vi "Actor Core.vi"(8 "error in":errorcluster, 11 "Main Display in":refnum<class "Main Display.lvclass">) -> (0 "error out":errorcluster, 3 "Actor out":refnum<class "Actor.lvclass">)   [LabVIEW 2016, in "Assert API Components.lvlib" / "Assert Display.lvlib" / "Main Display.lvlib" / "Main Display.lvclass"]
doc: "(<B>Filename</B>: Actor Framework.lvlib:Actor.lvclass:Actor Core.vi)\n\nReceives messages to the actor, reacts to them, and initiates any error handling that may shut the actor down.\n\nDescendant classes may override this VI to append parallel tasks for the actor to complete while it handles messages. Overrides use the Call Parent Method node."
uses:
  Main Display.lvclass
  C:/Program Files (x86)/National Instruments/LabVIEW 2016/vi.lib/ActorFramework/Actor/Actor.lvclass
  D:/Work/Projects/actor_assert_api/Base UI Component/Base UI Component/Base UI Component.lvclass
  D:/Work/Projects/actor_assert_api/Base UI Actor/Base UI Actor/Base UI Actor.lvclass
  <vilib>/ActorFramework/Actor/Actor.lvclass
  Timing Engine/Timing Engine/Timing Engine.lvclass
  Main Display.lvclass/Main Display.ctl
  Base UI Actor/Base UI Actor/Base UI Actor.lvclass/Base UI Actor.ctl
  Base UI Component/Base UI Component/Base UI Component.lvclass/Base UI Component.ctl
  <vilib>/ActorFramework/Actor/Actor.lvclass/Actor.ctl
  <vilib>/ActorFramework/Message Enqueuer/Message Enqueuer.lvclass/Message Enqueuer.ctl
  Action Configuration.ctl
  Actions.ctl
  Main Display Messages/Do Action Msg/Do Action Msg.lvclass/Do Action Msg.ctl
  <vilib>/ActorFramework/Message Enqueuer/Init from Existing Queue.vi
  <vilib>/ActorFramework/Message Enqueuer/Enqueue.vi
  Main Display Messages/Do Action Msg/Do Action Msg.lvclass
  C:/Program Files (x86)/National Instruments/LabVIEW 2016/vi.lib/ActorFramework/Message/Message.lvclass
  <vilib>/Utility/LVClass/Get LV Class Name.vi
  <resource>/AFDebug/Generate Trace for Message.vi
  <vilib>/ActorFramework/Message Priority Queue/Priority Enqueue.vi
  <vilib>/ActorFramework/Message Enqueuer/Message Enqueuer.lvclass
  Base UI Component/Base UI Component/Base UI Component.lvclass
  Right Click Menu Actions/RCM_Actions.lvclass
  Base UI Actor/Base UI Actor/Base UI Actor.lvclass
panel:
  in  "Settings":bool
  in  "Main":bool
  out "Tab Control":enum32{"Display", "Settings"}(tab)
  in  "Assert Display Data":i32(listbox)
  in  "Display Update Period":i32(slide)=1000 min=10 max=10000 scale=10.0..10000.0
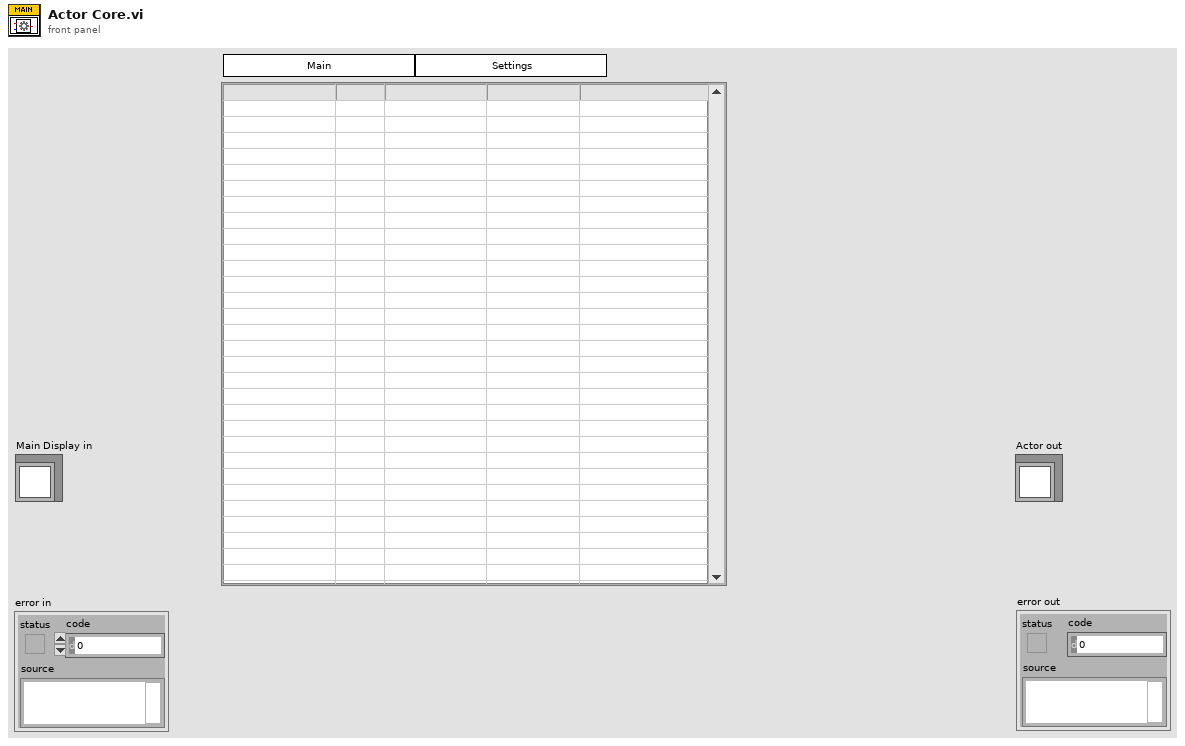
[diagram p1: front panel]
types:
  T1 = typedef "Assert API Components.lvlib/Assert Display.lvlib/Main Display.lvlib/Main Display.lvclass/Actions.ctl" = enum16{"Update Column Headers", "Update Timeout"}
  T2 = typedef "Assert API Components.lvlib/Assert Display.lvlib/Main Display.lvlib/Main Display.lvclass/Action Configuration.ctl" = cluster{"Action":T1, "Configuration":variant}
  T3 = typedef "LVPoint32TypeDef.ctl" = cluster{"Horizontal":i32, "Vertical":i32}
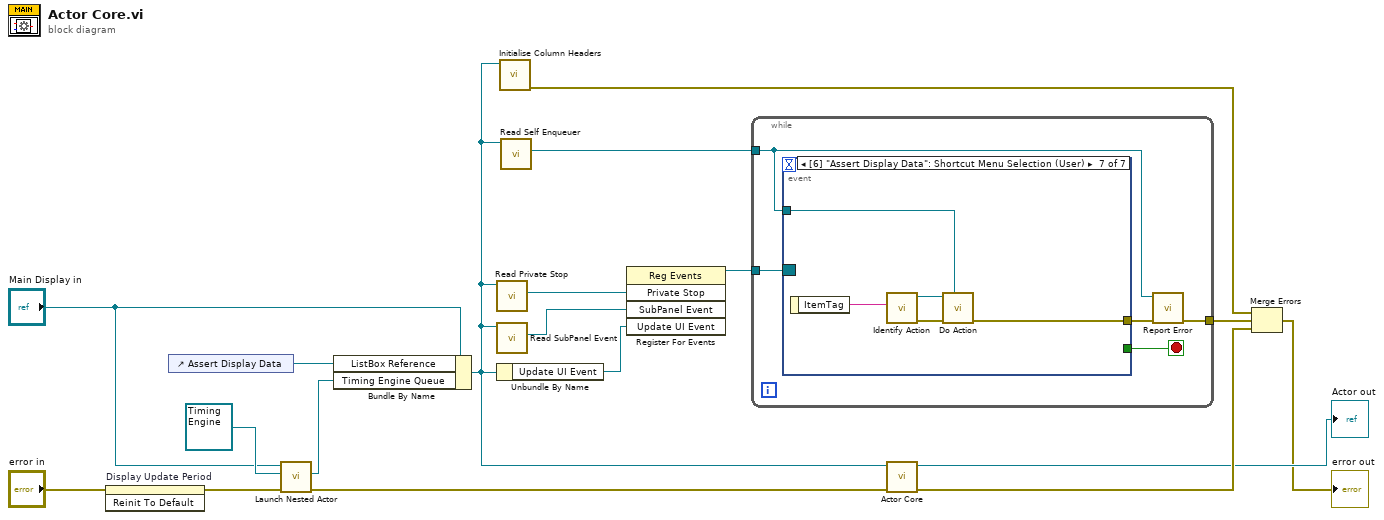
[diagram p0: block diagram]
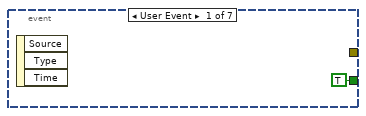
[diagram p2: hidden frame]
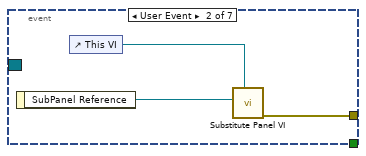
[diagram p3: hidden frame]
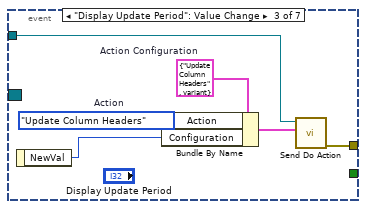
[diagram p4: hidden frame]
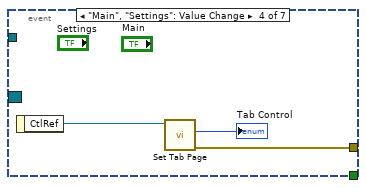
[diagram p5: hidden frame]
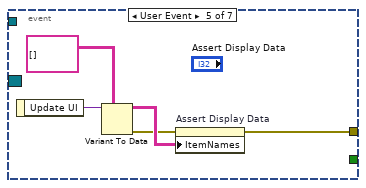
[diagram p6: hidden frame]
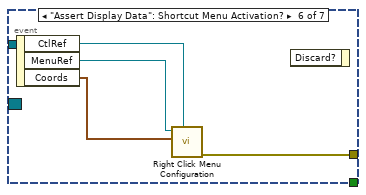
[diagram p7: hidden frame]
diagram:
  n1 = invoke on="Display Update Period" class="Slide (strict)" method="Reinit To Default"(error in="error in") -> (error out=w5:errorcluster)  [unwired: 2 in, 2 out]
  n2 = control-ref of="Assert Display Data"() -> (w1:refnum<vi>)
  n3 = call <vilib>:"Launch Nested Actor.vi"("error in (no error)"=w5, "Nested Actor"=refnum<class "Timing Engine.lvclass"> refnum ("Assert Display.lvlib:Timing Engine.lvlib:Timing Engine.lvclass"), "Caller Actor in"="Main Display in") -> ("error out"=w9:errorcluster, "Nested Actor's Enqueuer"=w10:refnum<class "Message Enqueuer.lvclass">)  [unwired: 6 in, 1 out]
  n4 = Bundle By Name(cluster="Main Display in", "ListBox Reference"=w1, "Timing Engine Queue"=w10) -> (w3:refnum<class "Main Display.lvclass">)
  n5 = call "Read Private Stop.vi"("Base UI Actor in"=w3) -> ("Private Stop"=w16:refnum<user-event>)  [unwired: 10 in]
  n6 = call "Read SubPanel Event.vi"("Base UI Component in"=w3) -> ("SubPanel Event"=w15:refnum<user-event>)  [unwired: 10 in]
  n7 = Unbundle By Name(w3) -> ("Update UI Event"=w6:refnum<user-event>)
  n8 = call "Initialise Column Headers.vi"("Main Display in"=w3) -> ("error out"=w2:errorcluster)  [unwired: 10 in]
  n9 = call <vilib>:"Read Self Enqueuer.vi"("Actor"=w3) -> ("Self Enqueuer"=w4:refnum<class "Message Enqueuer.lvclass">)  [unwired: 10 in]
  n10 = register-events(w16, w15, w6) -> (reference out=w14:refnum<event-registration>)  [unwired: 2 in, 1 out]
  n11 = while {
    tunnel: w14 -> [w23]
    tunnel: [w20] -> w12
    tunnel: w4 -> [w19]
    stop <- w21 stop-if-true
    n12 = event shown="[6] \"Assert Display Data\": Shortcut Menu Selection (User)" {
      selector: w23 -> [_ _ _ _ _ _ _]
      dyn-events: _ -> [_ _ _ _ _ _ _]
      timeout: _ -> [_ _ _ _ _ _ _]
      tunnel: [_ w27 w32 w35 w37 w45 w47] -> w22
      tunnel: [TRUE _ _ _ _ _ _] -> w21
      tunnel: w19 -> [_ _ w33 _ _ _ w46]
      event User Event {
        n13 = event-data() -> ()  [unwired: 1 in, 3 out]
      }
      event User Event {
        n14 = event-data() -> ("SubPanel Reference"=w26:refnum<vi>)  [unwired: 1 in]
        n15 = control-ref of="This VI"() -> (w25:refnum<vi>)
        n16 = call "Substitute Panel VI.vi"("VI Reference"=w25, "SubPanel Reference"=w26) -> ("error out"=w27:errorcluster)  [unwired: 9 in]
      }
      event "Display Update Period": Value Change {
        w29 = Actions."Update Column Headers"  # Action
        w31 = T2 {"Action"=enum."Update Column Headers", "Configuration"=variant}  # Action Configuration
        n17 = event-data() -> ("NewVal"=w28:i32)  [unwired: 1 in]
        n18 = Bundle By Name(cluster=w31, "Action"=w29, "Configuration"=w28) -> (w30:T2)
        n19 = call "Send Do Action.vi"("Action Configuration"=w30, "Message Enqueuer"=w33) -> ("error out"=w32:errorcluster)  [unwired: 8 in, 1 out]
      }
      event "Main", "Settings": Value Change {
        n20 = event-data() -> ("CtlRef"=w36:refnum<vi>)  [unwired: 1 in]
        n21 = call "Set Tab Page.vi"("Control Reference in"=w36) -> ("error out"=w35:errorcluster, "Tab Control"=→"Tab Control":enum32{"Display", "Settings"})  [unwired: 9 in]
      }
      event User Event {
        n22 = event-data() -> ("Update UI"=w41:variant)  [unwired: 1 in]
        n23 = Variant To Data(type=string[][] [], Variant=w41) -> (data=w39:string[][], error out=w38:errorcluster)  [unwired: 1 in]
        n24 = property on="Assert Display Data" class="MCListbox (strict)"(error in=w38, "ItemNames"=w39) -> (error out=w37:errorcluster)  [unwired: 1 in, 1 out]
      }
      event "Assert Display Data": Shortcut Menu Activation? {
        n25 = event-data() -> ("CtlRef"=w42:refnum<vi>, "MenuRef"=w43:refnum<k9>, "Coords"=w44:T3)  [unwired: 1 in]
        n26 = call "Right Click Menu Configuration.vi"("MCListbox Refnum"=w42, "Coords"=w44, "MenuRef"=w43) -> ("error out"=w45:errorcluster)  [unwired: 8 in]
        n27 = event-data() -> ()  [unwired: 2 in, 1 out]
      }
      event "Assert Display Data": Shortcut Menu Selection (User) {
        n28 = event-data() -> ("ItemTag"=w50:string)  [unwired: 1 in]
        n29 = call "Identify Action.vi"("Item Tag"=w50) -> ("error out"=w48:errorcluster, "RCM_Actions out"=w49:refnum<class "RCM_Actions.lvclass">)  [unwired: 9 in]
        n30 = call-dynamic "Do Action.vi"("Self Enqueuer"=w46, "error in (no error)"=w48, "RCM_Actions in"=w49) -> ("error out"=w47:errorcluster)  [unwired: 8 in]
      }
    }
    n31 = call "Report Error.vi"("error in (no error)"=w22, "Self Enqueuer"=w19) -> ("error out"=w20:errorcluster)  [unwired: 9 in]
  }
  n32 = call-parent "Actor Core.vi"("error in"=w9, "Actor in"=w3) -> ("error out"=w18:errorcluster, "Actor out"=→"Actor out":refnum<class "Actor.lvclass">)  [unwired: 8 in]
  n33 = Merge Errors(w2, w12, w18) -> (→"error out":errorcluster)
